vi "Create Logger.vi"(8 "error in (no error)":errorcluster, 10 "Name":string, 11 "Registry in":refnum<class "Registry.lvclass">) -> (0 "error out":errorcluster, 2 "Logger out":refnum<class "Logger.lvclass">, 3 "Registry out":refnum<class "Registry.lvclass">)   [LabVIEW 2025, in "LV Logging.lvlib" / "Registry.lvclass"]
uses:
  Registry.lvclass
  Logger/Logger.lvclass
  Logger/Logger.lvclass/Logger.ctl
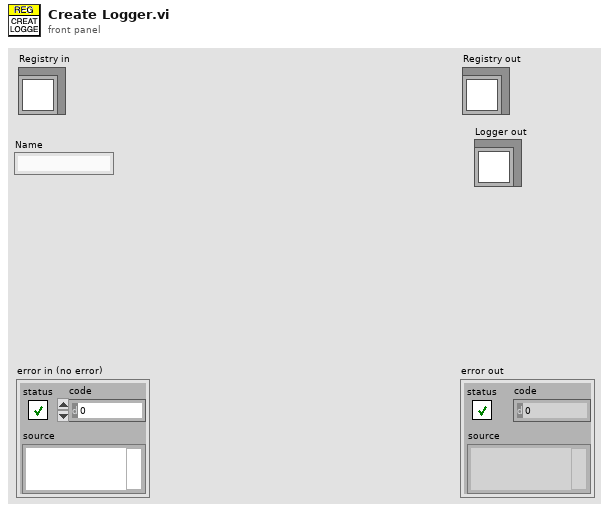
[diagram p1: front panel]
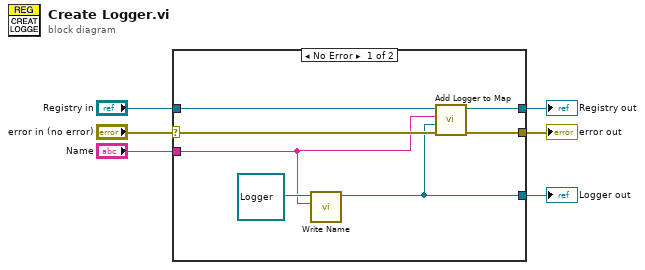
[diagram p0: block diagram]
diagram:
  n1 = case shown="No Error" "error in (no error)" {
    selector: "error in (no error)" -> [w10 w15]
    tunnel: [w9 w15] -> w5
    tunnel: [w11 w14] -> w3
    tunnel: "Registry in" -> [w12 w14]
    tunnel: "Name" -> [w8 _]
    tunnel: [w7 _] -> w1
    frame No Error {
      n2 = call "Write Name.vi"("Name"=w8, "Logger in"=refnum<class "Logger.lvclass"> refnum ("LV Logging.lvlib:Logger.lvclass")) -> ("Logger out"=w7:refnum<class "Logger.lvclass">)  [unwired: 8 in, 1 out]
      n3 = call "Add Logger to Map.vi"("error in (no error)"=w10, "Logger"=w7, "Name"=w8, "Registry in"=w12) -> ("error out"=w9:errorcluster, "Registry out"=w11:refnum<class "Registry.lvclass">)  [unwired: 6 in]
    }
    frame Error {
    }
  }
  "error out" <- w5
  "Registry out" <- w3
  "Logger out" <- w1
